vi "流程批量写入.vi"(10 "简易流程路径":path, 11 "添加的路径":path caption="测试流程路径") -> ()   [LabVIEW 2016, in "斯坦道氨氮.lvlib"]
uses:
  <vilib>/Utility/miscctls.llb/LVPointTypeDef.ctl
panel:
  in  "校验":bool
  in  "选项卡控件":enum32{"测试流程", "简易流程"}(tab)
  in  "一键写入":bool
  in  "量程下拉列表":enum16{"低量程", "高量程"}(ring)
  in  "测量模式":T1(ring)
  in  "简易流程":u16(ring)
  in  "一键写入 2":bool=TRUE
  in  "关闭":bool
  out "字符串":string
  in  "写入":bool
  in  "参数下拉列表":u16(ring) items=["总氮"=2, "总磷"=1]
  # "请选择要写入的流程"
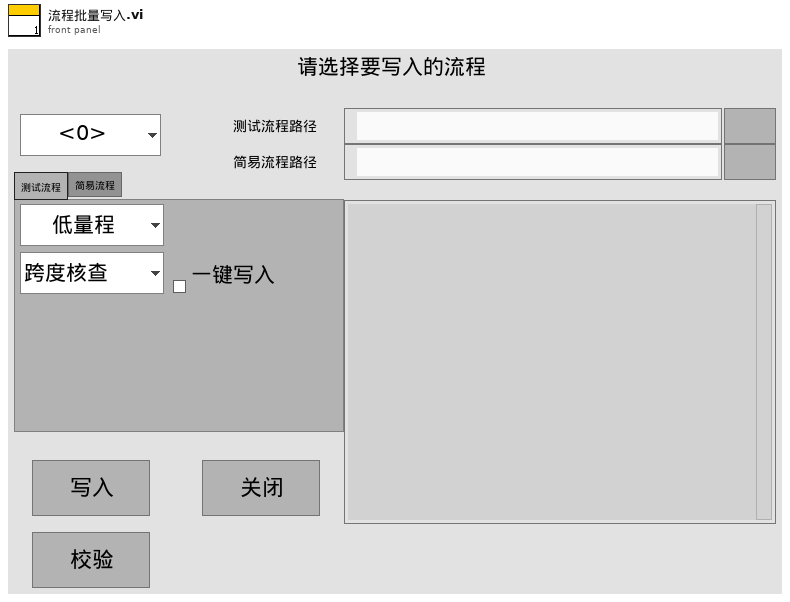
[diagram p1: front panel]
types:
  T1 = enum16{"跨度核查", "水样测量", "零点核查", "标样核查", "加标回收", "快捷测试", "空白校准", "标样校准"}
  T2 = typedef "LVPointTypeDef.ctl" = cluster{"Horizontal":i16, "Vertical":i16}
  T3 = typedef "LVStringsAndValuesArrayTypeDef_U16.ctl" = cluster{"String":string, "Value":u16}[]
  T4 = typedef "操作日志字段定义.ctl" = cluster{"时间":timestamp, "参数":string, "日志信息":string, "流程参数":string}
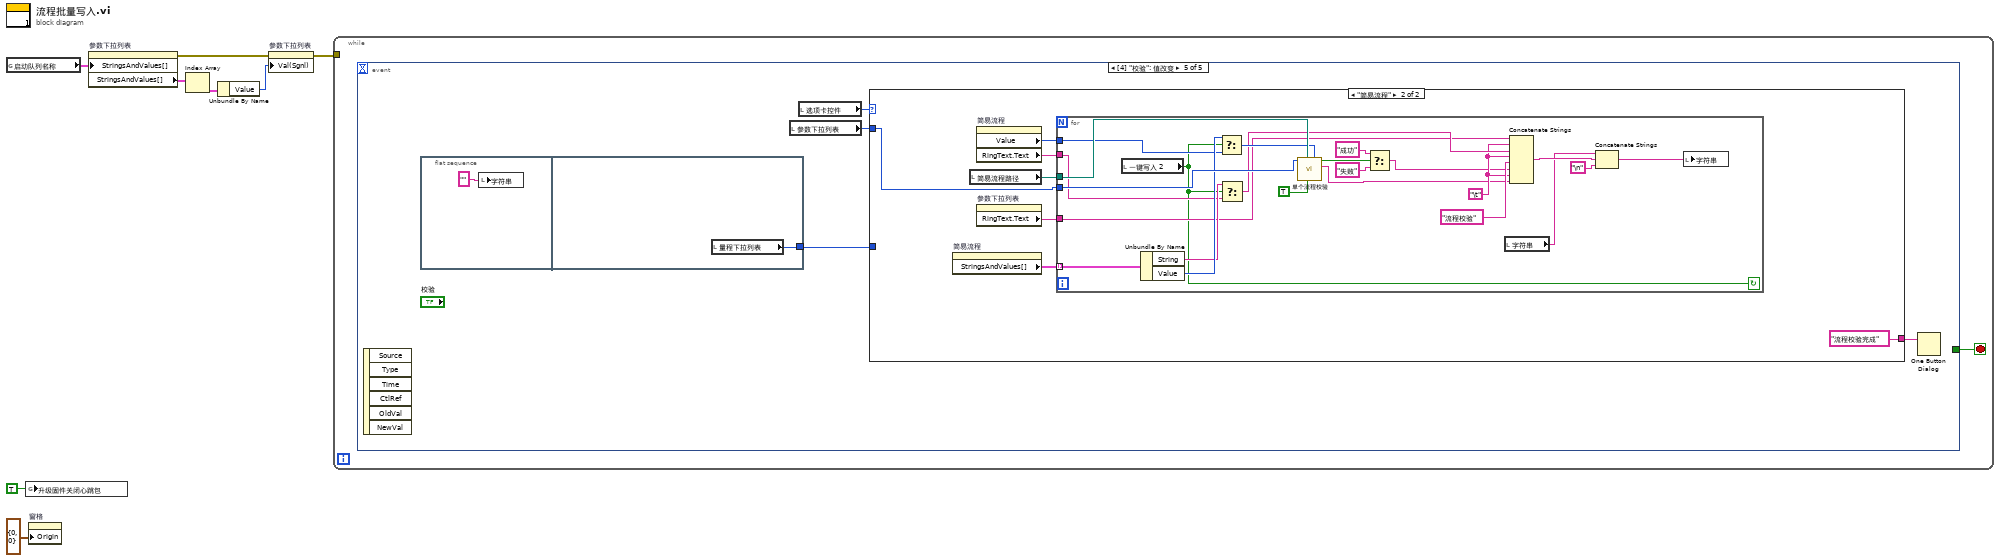
[diagram p0: block diagram]
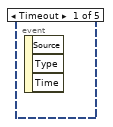
[diagram p2: hidden frame]
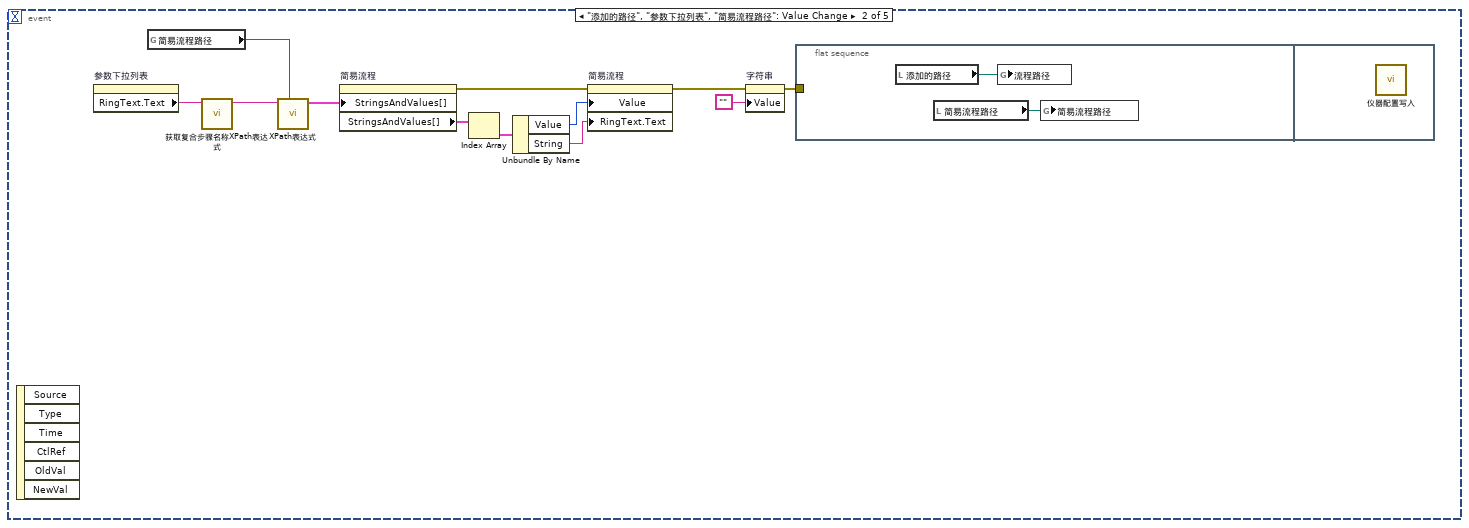
[diagram p3: hidden frame]
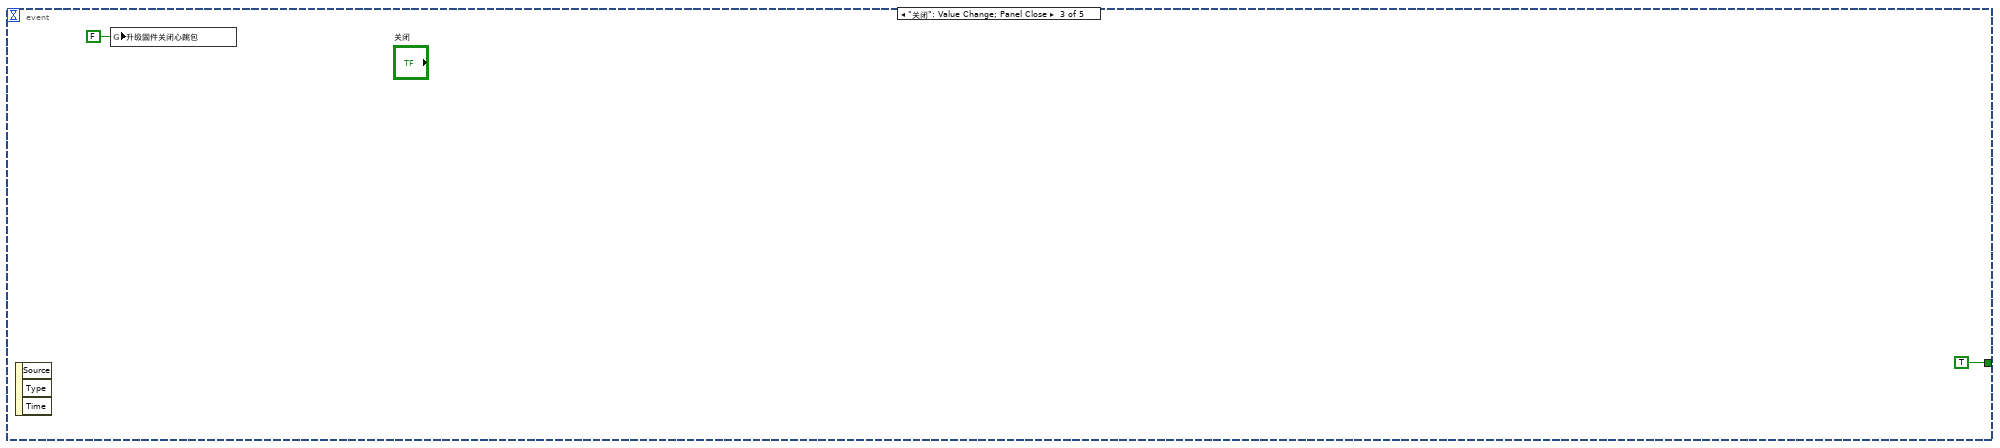
[diagram p4: hidden frame]
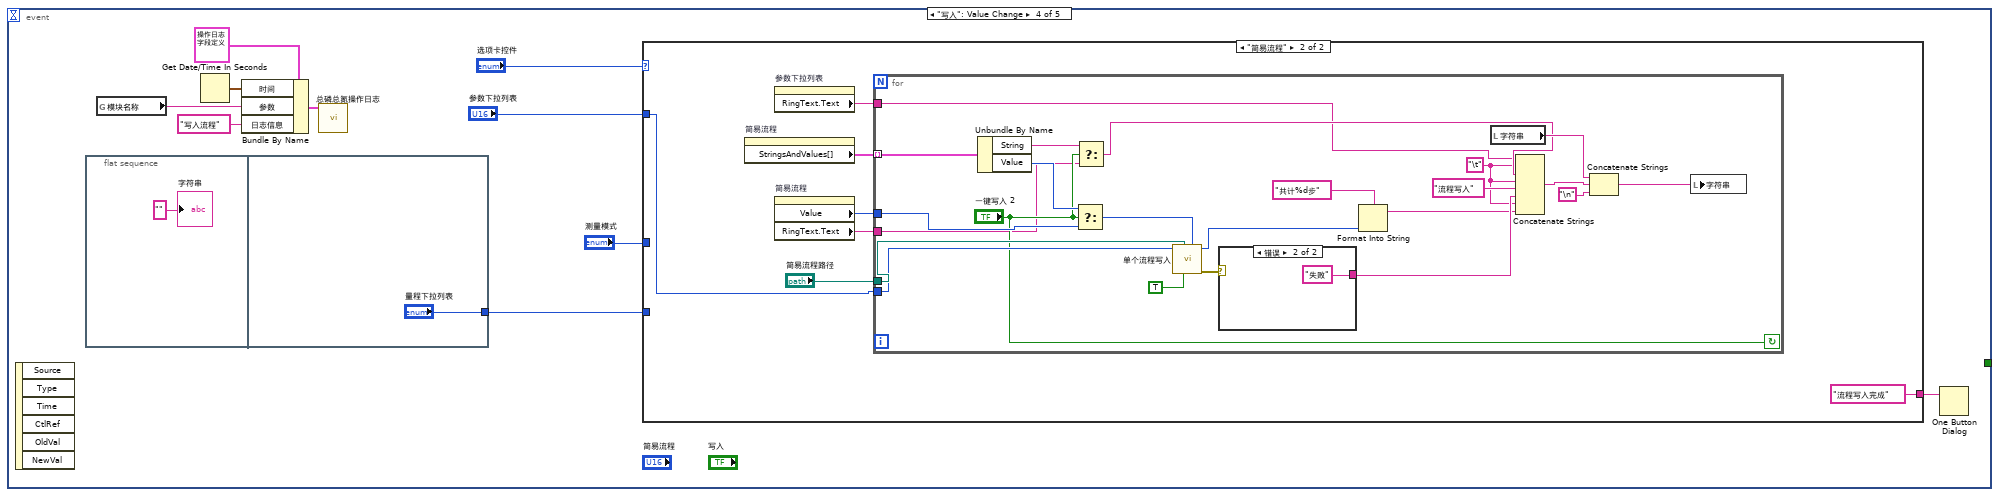
[diagram p5: hidden frame]
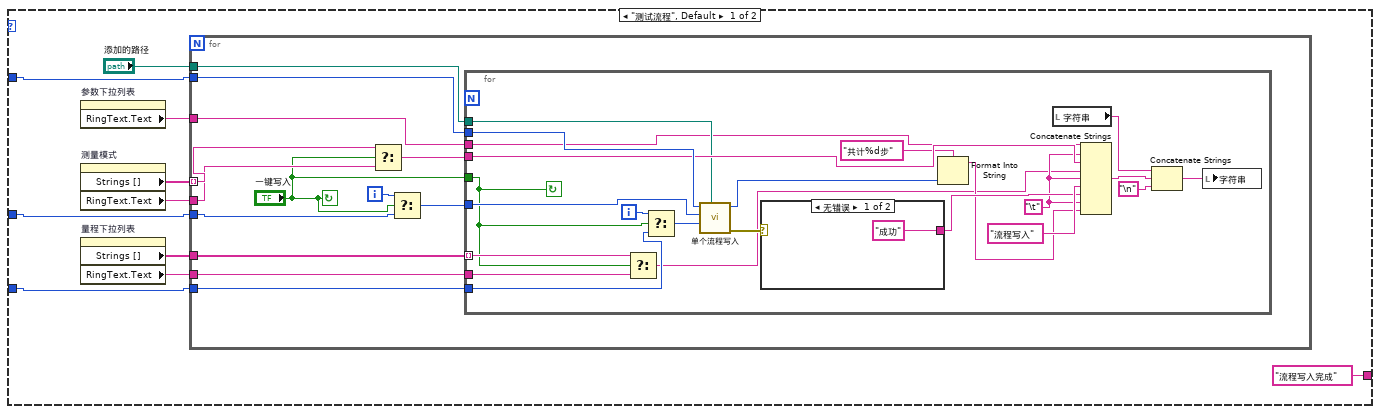
[diagram p6: hidden frame]
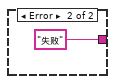
[diagram p7: hidden frame]
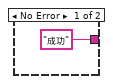
[diagram p8: hidden frame]
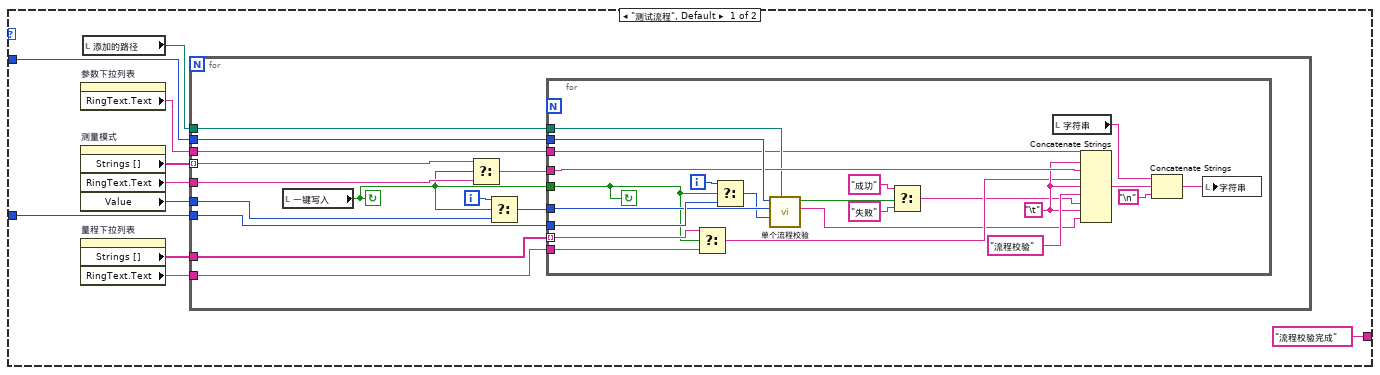
[diagram p9: hidden frame]
diagram:
  n1 = global read "model config var.vi" "启动队列名称"() -> (w7:cluster{"String":string, "Value":u16}[])
  n2 = global write "VAR总磷总氮全局变量.vi" "升级固件关闭心跳包"(TRUE ("升级固件关闭心跳包")) -> ()
  n3 = property on="窗格" class="Pane"("Origin"=T2 {"Horizontal"=0, "Vertical"=0} ("原点")) -> ()  [unwired: 2 in, 2 out]
  n4 = property on="参数下拉列表" class="Ring (严格)"("StringsAndValues[]"=w7) -> (error out=w6:errorcluster, "StringsAndValues[]"=w5:T3)  [unwired: 2 in, 1 out]
  n5 = Index Array(array=w5) -> (element=w4:cluster{"String":string, "Value":u16})  [unwired: 1 in]
  n6 = Unbundle By Name(w4) -> ("Value"=w3:u16)
  n7 = property on="参数下拉列表" class="Ring (严格)"(error in=w6, "Val(Sgnl)"=w3) -> (error out=w2:errorcluster)  [unwired: 1 in, 1 out]
  n8 = while {
    tunnel: w2 -> [_]
    stop <- w9 stop-if-true
    n9 = event shown="[4] \"校验\": 值改变" {
      selector: _ -> [_ _ _ _ _]
      dyn-events: _ -> [_ _ _ _ _]
      timeout: _ -> [_ _ _ _ _]
      tunnel: [_ _ TRUE _ _] -> w9
      event Timeout {
        n10 = event-data() -> ()  [unwired: 1 in, 3 out]
      }
      event "添加的路径", "参数下拉列表", "简易流程路径": Value Change {
        n11 = event-data() -> ()  [unwired: 1 in, 6 out]
        n12 = property on="参数下拉列表" class="Ring (严格)"() -> ("RingText.Text"=w11:string)  [unwired: 2 in, 2 out]
        n13 = global read "总磷总氮断电保存全局变量.vi" "简易流程路径"() -> (w12:path)
        n14 = call "获取复合步骤名称XPath表达式.vi"("查询参数"=w11) -> ("Union"=w13:string)  [unwired: 10 in]
        n15 = call "XPath表达式.vi"("添加的路径"=w12, "XPath expression"=w13) -> ("数组"=w10:cluster{string, i32}[])  [unwired: 9 in]
        n16 = property on="简易流程" class="Ring (严格)"("StringsAndValues[]"=w10) -> (error out=w20:errorcluster, "StringsAndValues[]"=w18:T3)  [unwired: 2 in, 1 out]
        n17 = Index Array(array=w18) -> (element=w17:cluster{"String":string, "Value":u16})  [unwired: 1 in]
        n18 = Unbundle By Name(w17) -> ("Value"=w16:u16, "String"=w14:string)
        n19 = property on="简易流程" class="Ring (严格)"(error in=w20, "Value"=w16, "RingText.Text"=w14) -> (error out=w19:errorcluster)  [unwired: 1 in, 1 out]
        n20 = property on="字符串" class="Str"(error in=w19, "Value"="") -> (error out=w15:errorcluster)  [unwired: 1 in, 1 out]
        n21 = flat-sequence {
          tunnel: w15 -> [_]
          frame #0 {
            n22 = local read "添加的路径"() -> (w22:path)
            n23 = local read "简易流程路径"() -> (w23:path)
            n24 = global write "总磷总氮断电保存全局变量.vi" "流程路径"(w22) -> ()
            n25 = global write "总磷总氮断电保存全局变量.vi" "简易流程路径"(w23) -> ()
          }
          frame #1 {
            n26 = call "仪器配置写入.vi"() -> ()  [unwired: 11 in, 1 out]
          }
        }
      }
      event "关闭": Value Change; Panel Close {
        n27 = event-data() -> ()  [unwired: 1 in, 3 out]
        n28 = global write "VAR总磷总氮全局变量.vi" "升级固件关闭心跳包"(FALSE ("升级固件关闭心跳包")) -> ()
      }
      event "写入": Value Change {
        n29 = event-data() -> ()  [unwired: 1 in, 6 out]
        n30 = flat-sequence {
          tunnel: ["量程下拉列表"] -> w34
          frame #0 {
            "字符串" <- ""
          }
          frame #1 {
          }
        }
        n31 = global read "VAR总磷总氮全局变量.vi" "模块名称"() -> (w26:string)
        n32 = Get Date/Time In Seconds() -> (seconds since 1Jan1904=w28:timestamp)
        n33 = Bundle By Name(cluster=T4 {"时间"=timestamp(0 s since 1904-01-01), "参数"="", "日志信息"="", "流程参数"=""} ("data in"), "时间"=w28, "参数"=w26, "日志信息"="写入流程") -> (w29:T4)
        n34 = call "总磷总氮操作日志.vi"("data in"=w29) -> ()  [unwired: 10 in, 1 out]
        n35 = case shown="\"简易流程\"" "选项卡控件" {
          tunnel: "参数下拉列表" -> [w43 w90]
          tunnel: w34 -> [w44 _]
          tunnel: ["流程写入完成" ("消息") "流程写入完成" ("消息")] -> w32
          tunnel: "测量模式" -> [w41 _]
          frame "测试流程", Default {
            n36 = property on="参数下拉列表" class="Ring (严格)"() -> ("RingText.Text"=w38:string)  [unwired: 2 in, 2 out]
            n37 = property on="测量模式" class="Enum (严格)"() -> ("Strings []"=w42:string[], "RingText.Text"=w39:string)  [unwired: 2 in, 2 out]
            n38 = property on="量程下拉列表" class="Enum (严格)"() -> ("Strings []"=w36:string[], "RingText.Text"=w40:string)  [unwired: 2 in, 2 out]
            n39 = for {
              tunnel: w44 -> [w58]
              tunnel: w43 -> [w56]
              tunnel: w42 -> [w52] mode=indexing
              tunnel: w41 -> [w55]
              tunnel: w40 -> [w53]
              tunnel: w39 -> [w51]
              tunnel: "添加的路径" -> [w49]
              tunnel: w38 -> [w48]
              tunnel: w36 -> [w46]
              i -> [w57]
              stop <- "一键写入" continue-if-true
              n40 = Select(t=w52, s="一键写入", f=w51) -> (s? t:f=w50:string)
              n41 = Select(t=w57, s="一键写入", f=w55) -> (s? t:f=w54:i32)
              n42 = for {
                tunnel: w58 -> [w74]
                tunnel: w56 -> [w73]
                tunnel: w54 -> [w72]
                tunnel: w53 -> [w61]
                tunnel: w50 -> [w71]
                tunnel: w49 -> [w70]
                tunnel: w48 -> [w69]
                tunnel: "一键写入" -> [w59]
                tunnel: w46 -> [w62] mode=indexing
                i -> [w63]
                stop <- w59 continue-if-true
                w65 = "\t"
                n43 = Select(t=w62, s=w59, f=w61) -> (s? t:f=w60:string)
                n44 = Select(t=w63, s=w59, f=w74) -> (s? t:f=w64:i32)
                n45 = call "单个流程写入.vi"("添加的路径"=w70, "量程"=w64, "测量模式"=w72, "测量参数"=w73) -> ("error out"=w81:errorcluster, "大小"=w68:i32)  [unwired: 6 in]
                n46 = case shown="无错误" w81 {
                  tunnel: ["成功" "失败"] -> w78
                  frame No Error {
                  }
                  frame Error {
                  }
                }
                n47 = Format Into String(format string="共计%d步" ("格式字符串"), w68) -> (resulting string=w66:string)  [unwired: 2 in, 1 out]
                n48 = local read "字符串"() -> (w80:string)
                n49 = Concatenate Strings(w69, w65, w71, w60, w65, "流程写入", w78, w65, w66) -> (w77:string)
                n50 = Concatenate Strings(w80, w77, "\n") -> (w75:string)
                n51 = local write "字符串"(w75) -> ()
              }
            }
          }
          frame "简易流程" {
            n52 = property on="简易流程" class="Ring (严格)"() -> ("StringsAndValues[]"=w89:T3)  [unwired: 2 in, 2 out]
            n53 = property on="参数下拉列表" class="Ring (严格)"() -> ("RingText.Text"=w84:string)  [unwired: 2 in, 2 out]
            n54 = property on="简易流程" class="Ring (严格)"() -> ("Value"=w87:u16, "RingText.Text"=w86:string)  [unwired: 2 in, 2 out]
            n55 = for {
              tunnel: w89 -> [w103] mode=indexing
              tunnel: "简易流程路径" -> [w106]
              tunnel: w90 -> [w105]
              tunnel: w87 -> [w100]
              tunnel: w86 -> [w97]
              tunnel: w84 -> [w91]
              stop <- "一键写入 2" continue-if-true
              w92 = "\t"
              n56 = Unbundle By Name(w103) -> ("String"=w98:string, "Value"=w102:u16)
              n57 = Select(t=w102, s="一键写入 2", f=w100) -> (s? t:f=w101:u16)
              n58 = Select(t=w98, s="一键写入 2", f=w97) -> (s? t:f=w96:string)
              n59 = call "单个流程写入.vi"("简易流程Id"=w101, "是否是简易流程"=TRUE, "添加的路径"=w106, "测量参数"=w105) -> ("error out"=w113:errorcluster, "大小"=w95:i32)  [unwired: 6 in]
              n60 = case shown="错误" w113 {
                tunnel: ["成功" "失败"] -> w110
                frame No Error {
                }
                frame Error {
                }
              }
              n61 = Format Into String(format string="共计%d步" ("格式字符串"), w95) -> (resulting string=w93:string)  [unwired: 2 in, 1 out]
              n62 = local read "字符串"() -> (w112:string)
              n63 = Concatenate Strings(w91, w92, w96, w92, "流程写入", w110, w92, w93) -> (w109:string)
              n64 = Concatenate Strings(w112, w109, "\n") -> (w107:string)
              n65 = local write "字符串"(w107) -> ()
            }
          }
        }
        n66 = One Button Dialog(message=w32) -> ()  [unwired: 1 in, 1 out]
      }
      event "校验": Value Change {
        n67 = event-data() -> ()  [unwired: 1 in, 6 out]
        n68 = flat-sequence {
          tunnel: [w199] -> w121
          frame #0 {
            n69 = local write "字符串"("") -> ()
          }
          frame #1 {
            n70 = local read "量程下拉列表"() -> (w199:enum16{"低量程", "高量程"})
          }
        }
        n71 = local read "参数下拉列表"() -> (w118:u16)
        n72 = local read "选项卡控件"() -> (w119:enum32{"测试流程", "简易流程"})
        n73 = case shown="\"简易流程\"" w119 {
          tunnel: w118 -> [w129 w174]
          tunnel: w121 -> [w130 _]
          tunnel: ["流程校验完成" ("消息") "流程校验完成" ("消息")] -> w120
          frame "测试流程", Default {
            n74 = property on="参数下拉列表" class="Ring (严格)"() -> ("RingText.Text"=w125:string)  [unwired: 2 in, 2 out]
            n75 = property on="测量模式" class="Enum (严格)"() -> ("Strings []"=w128:string[], "RingText.Text"=w126:string, "Value"=w122:T1)  [unwired: 2 in, 2 out]
            n76 = property on="量程下拉列表" class="Enum (严格)"() -> ("Strings []"=w124:string[], "RingText.Text"=w127:string)  [unwired: 2 in, 2 out]
            n77 = local read "添加的路径"() -> (w123:path)
            n78 = for {
              tunnel: w130 -> [w144]
              tunnel: w129 -> [w142]
              tunnel: w128 -> [w138] mode=indexing
              tunnel: w122 -> [w141]
              tunnel: w127 -> [w139]
              tunnel: w126 -> [w137]
              tunnel: w123 -> [w135]
              tunnel: w125 -> [w134]
              tunnel: w124 -> [w133]
              i -> [w143]
              stop <- w132 continue-if-true
              n79 = local read "一键写入"() -> (w132:bool)
              n80 = Select(t=w138, s=w132, f=w137) -> (s? t:f=w136:string)
              n81 = Select(t=w143, s=w132, f=w141) -> (s? t:f=w140:i32)
              n82 = for {
                tunnel: w144 -> [w164]
                tunnel: w142 -> [w163]
                tunnel: w140 -> [w162]
                tunnel: w139 -> [w154]
                tunnel: w136 -> [w161]
                tunnel: w135 -> [w160]
                tunnel: w134 -> [w159]
                tunnel: w132 -> [w145]
                tunnel: w133 -> [w155] mode=indexing
                i -> [w156]
                stop <- w145 continue-if-true
                w158 = "\t"
                n83 = Select(t=w155, s=w145, f=w154) -> (s? t:f=w153:string)
                n84 = Select(t=w156, s=w145, f=w164) -> (s? t:f=w157:i32)
                n85 = call "单个流程校验.vi"("添加的路径"=w160, "量程"=w157, "测量模式"=w162, "测量参数"=w163) -> ("结果字符串"=w146:string, "check？"=w147:bool)  [unwired: 5 in, 1 out]
                n86 = Select(t="成功", s=w147, f="失败") -> (s? t:f=w148:string)
                n87 = local read "字符串"() -> (w152:string)
                n88 = Concatenate Strings(w159, w158, w161, w153, w158, "流程校验", w148, w158, w146) -> (w166:string)
                n89 = Concatenate Strings(w152, w166, "\n") -> (w151:string)
                n90 = local write "字符串"(w151) -> ()
              }
            }
          }
          frame "简易流程" {
            n91 = property on="简易流程" class="Ring (严格)"() -> ("StringsAndValues[]"=w173:T3)  [unwired: 2 in, 2 out]
            n92 = local read "简易流程路径"() -> (w168:path)
            n93 = property on="简易流程" class="Ring (严格)"() -> ("Value"=w171:u16, "RingText.Text"=w170:string)  [unwired: 2 in, 2 out]
            n94 = property on="参数下拉列表" class="Ring (严格)"() -> ("RingText.Text"=w169:string)  [unwired: 2 in, 2 out]
            n95 = for {
              tunnel: w173 -> [w191] mode=indexing
              tunnel: w168 -> [w194]
              tunnel: w174 -> [w193]
              tunnel: w171 -> [w188]
              tunnel: w170 -> [w186]
              tunnel: w169 -> [w183]
              stop <- w182 continue-if-true
              w184 = "\t"
              n96 = local read "一键写入 2"() -> (w182:bool)
              n97 = Unbundle By Name(w191) -> ("String"=w187:string, "Value"=w190:u16)
              n98 = Select(t=w190, s=w182, f=w188) -> (s? t:f=w189:u16)
              n99 = Select(t=w187, s=w182, f=w186) -> (s? t:f=w185:string)
              n100 = call "单个流程校验.vi"("简易流程Id"=w189, "是否是简易流程"=TRUE, "添加的路径"=w194, "测量参数"=w193) -> ("结果字符串"=w175:string, "check？"=w176:bool)  [unwired: 5 in, 1 out]
              n101 = Select(t="成功", s=w176, f="失败") -> (s? t:f=w177:string)
              n102 = local read "字符串"() -> (w181:string)
              n103 = Concatenate Strings(w183, w184, w185, w184, "流程校验", w177, w184, w175) -> (w196:string)
              n104 = Concatenate Strings(w181, w196, "\n") -> (w180:string)
              n105 = local write "字符串"(w180) -> ()
            }
          }
        }
        n106 = One Button Dialog(message=w120) -> ()  [unwired: 1 in, 1 out]
      }
    }
  }
